vi "Set_Radio_Device_Serial_Name.vi"(8 "error in (no error)":errorcluster, 9 "Serial Name":string="332DC15", 10 "Cellular Technology":T2, 11 "Base Station":T1) -> (0 "error out":errorcluster, 3 "Output String":string)   [LabVIEW 2021]
uses:
  Controls/Cellular_Technology.ctl
  Controls/Base_Station_Emulator.ctl
  Controls/TCP_FGV.ctl
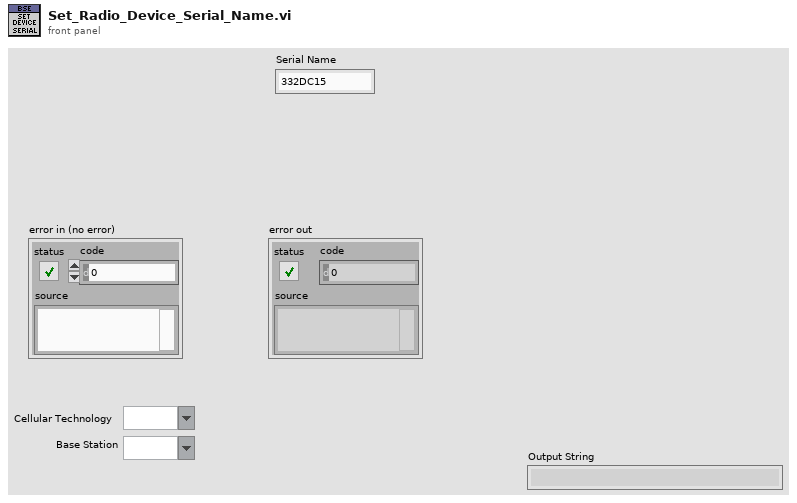
[diagram p1: front panel]
types:
  T1 = typedef "Base_Station_Emulator.ctl" = string
  T2 = typedef "Cellular_Technology.ctl" = string
  T3 = typedef "TCP_FGV.ctl" = enum16{"Open", "Read", "Write", "Close"}
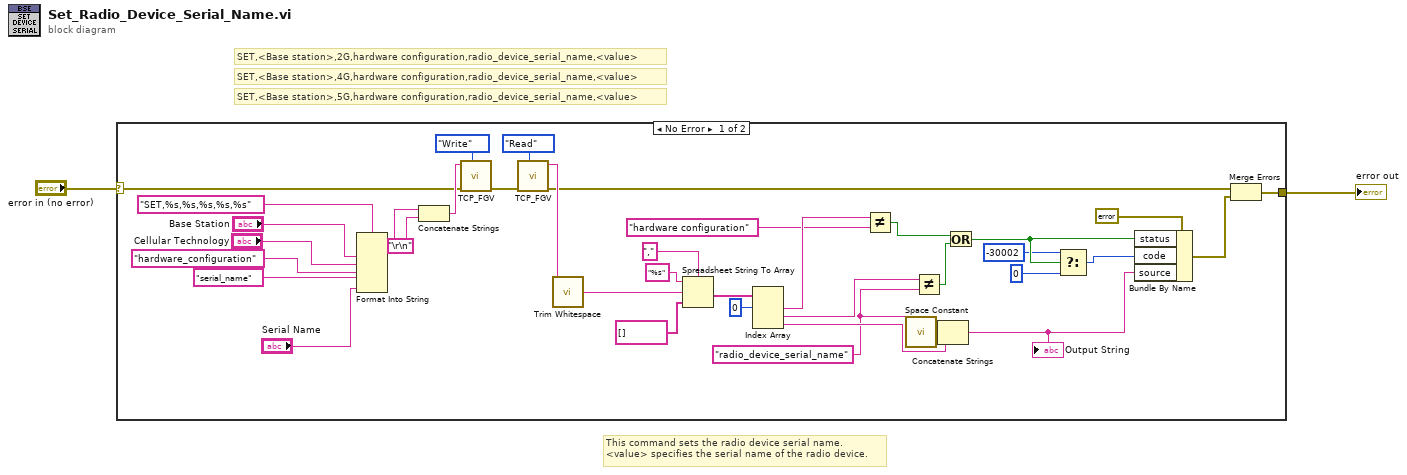
[diagram p0: block diagram]
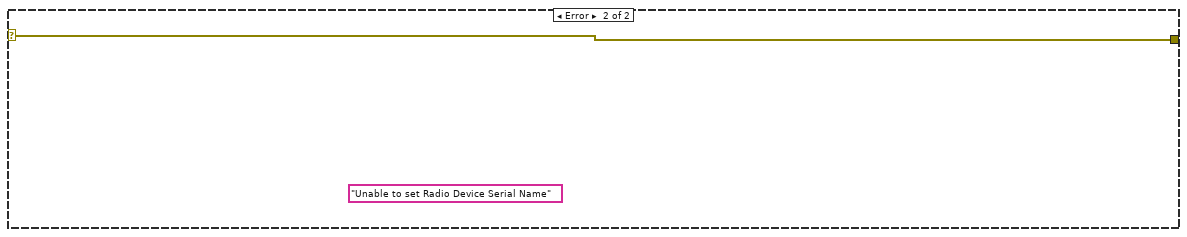
[diagram p2: hidden frame]
diagram:
  # "This command sets the radio device serial name.   \n<value> specifies the serial name of the radio device."
  # "SET,<Base station>,5G,hardware configuration,radio_device_serial_name,<value>"
  # "SET,<Base station>,4G,hardware configuration,radio_device_serial_name,<value>"
  # "SET,<Base station>,2G,hardware configuration,radio_device_serial_name,<value>"
  n1 = case shown="No Error" "error in (no error)" {
    selector: "error in (no error)" -> [w4 w40]
    tunnel: [w17 w40] -> w1
    frame No Error {
      w10 = "radio_device_serial_name"
      n2 = Format Into String(format string="SET,%s,%s,%s,%s,%s", "Base Station", "Cellular Technology", "hardware_configuration", "serial_name", "Serial Name") -> (resulting string=w6:string)  [unwired: 2 in, 1 out]
      n3 = Concatenate Strings(w6, "\r\n") -> (w5:string)
      n4 = call "TCP_FGV.vi"("Command"=w5, "error in (no error)"=w4, "Operation"=TCP_FGV."Write") -> ("error out"=w34:errorcluster)  [unwired: 6 in, 1 out]
      n5 = call "TCP_FGV.vi"("error in (no error)"=w34, "Operation"=TCP_FGV."Read") -> ("Data Out"=w18:string, "error out"=w16:errorcluster)  [unwired: 7 in]
      n6 = call <vilib>:"Trim Whitespace.vi"("string"=w18) -> ("trimmed string"=w31:string)  [unwired: 1 in]
      n7 = Spreadsheet String To Array(delimiter (Tab)=",", format string="%s", spreadsheet string=w31, array type (2D Dbl)=string[] []) -> (array=w27:string[])
      n8 = Index Array(array=w27, index #1=0 ("index")) -> (element #1=w28:string, element #2=w14:string, element #3=w11:string)  [unwired: 2 in]
      n9 = Not Equal?(x=w28, y="hardware configuration" ("format string")) -> (x != y?=w29:bool)
      n10 = call <vilib>:"Space Constant.vi"() -> ("String"=w12:string)
      n11 = Not Equal?(x=w14, y=w10) -> (x != y?=w30:bool)
      n12 = Concatenate Strings(w10, w12, w11) -> (w13:string)
      "Output String" <- w13
      n13 = Or(x=w29, y=w30) -> (x .or. y?=w32:bool)
      n14 = Select(t=-30002 ("code"), s=w32, f=0 ("code")) -> (s? t:f=w33:i32)
      n15 = Bundle By Name(cluster=errorcluster {"status"=FALSE, "code"=0, "source"=""} ("error constant"), "status"=w32, "code"=w33, "source"=w13) -> (w15:errorcluster)
      n16 = Merge Errors(w16, w15) -> (w17:errorcluster)
    }
    frame Error {
      (unwired) "Unable to set Radio Device Serial Name" ("source")
    }
  }
  "error out" <- w1
